vi "DialogRasterCompute.vi"(6 "Mode":bool, 7 "aparCfg in":refnum<class "aparCfg.lvclass">, 10 "Data File Name":string, 11 "Motion64.ini path":path=path "C:/Users/Public/Documents/UCAR/APAR Board Test/SupportFiles/Motion64.ini") -> (1 "Position Array":T1(array[cluster]), 2 "Data File Name out":string, 3 "Cancelled?":bool, 5 "aparCfg out":refnum<class "aparCfg.lvclass">)   [LabVIEW 2017]
doc: "Use this template to create a dialog box with event handling."
uses:
  Classes/VXMCfg/VXMCfg.lvclass
  Classes/aparCfg/aparCfg.lvclass
  <vilib>/Utility/file.llb/Read Delimited Spreadsheet (DBL).vi
panel:
  out "64ModuleConfigs":string[][](table) caption="Configurations for the 64 Modules"
  in  "Polarization":enum16{"Vertical", "Horizontal"}(ring)=enum."Horizontal"
  in  "RF In/Out":enum16{"Tx - RF In", "Rx - RF Out"}(ring)=enum."Rx - RF Out"
  out "Total Points":dbl
  out "TestZT":cluster{"Z mm":dbl, "Horizontal T deg":dbl}
  out "XY Graph for evaluation":cluster{dbl[], dbl[]}[](graph)
  in  "Nyquist, mm":i32=28 caption="Nyquist Sampling Interval, mm" min=1 max=64 step=1
  in  "calculate":bool
  in  "Window dimension":i32=42 caption="Synthetic Window, cm" min=1 max=64 step=1
  in  "Cancel":bool
  in  "OK":bool
  # "Define Raster Positions"
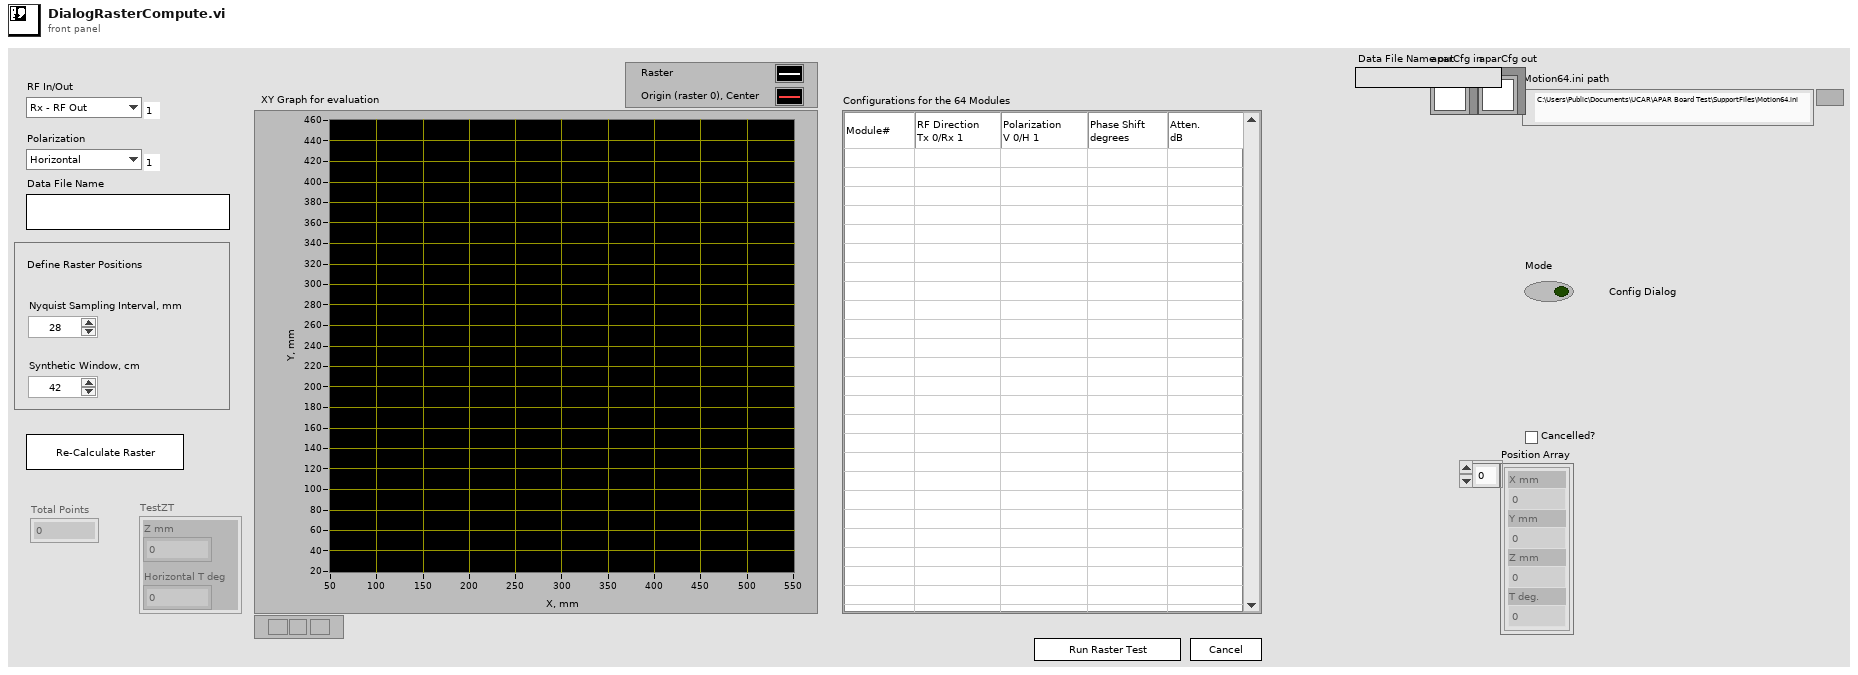
[diagram p1: front panel]
types:
  T1 = cluster{"X mm":dbl, "Y mm":dbl, "Z mm":dbl, "T deg.":dbl}[]
  T2 = typedef "rasterConfig.ctl" = cluster{"Nyquist, mm":dbl, "Window, cm":dbl, "Polarization, V0 H1":T3, "RF Direction Tx0":T4}
  T3 = typedef "PolarizationSelect.ctl" = enum16{"Vertical", "Horizontal"}
  T4 = typedef "RF Direction.ctl" = enum16{"Tx - RF In", "Rx - RF Out"}
  T5 = typedef "sub-syst.n.ctl" = cluster{"Addr":string, "Enable":bool, "X scale eng./step":dbl, "Y scale eng./step":dbl, "Z scale eng./step":dbl, "T scale eng./step":dbl, "X units":string, "Y units":string, "Z units":string, "T units":string, "X Jog":dbl, "Y Jog":dbl, "Z Jog":dbl, "T Jog":dbl, "VXM (1-4)":i32}
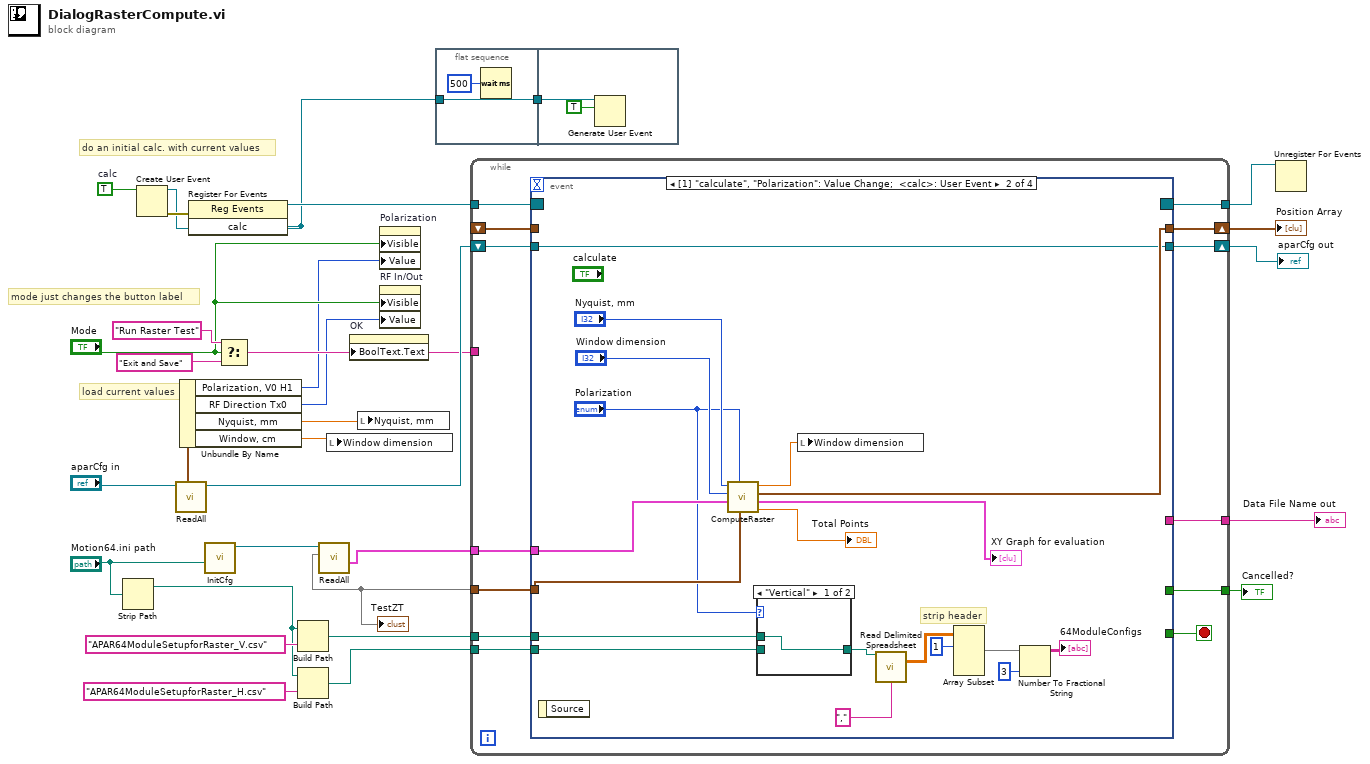
[diagram p0: block diagram]
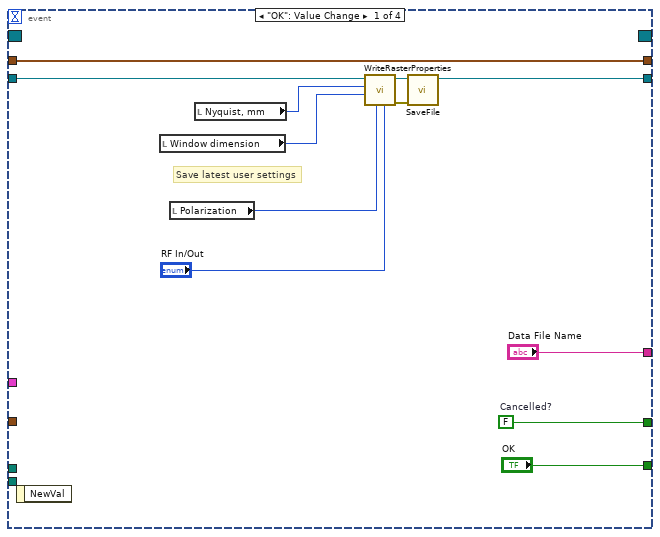
[diagram p2: hidden frame]
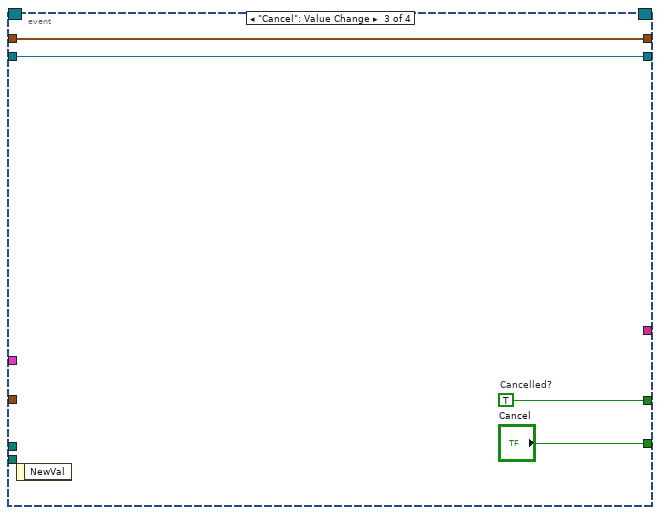
[diagram p4: hidden frame]
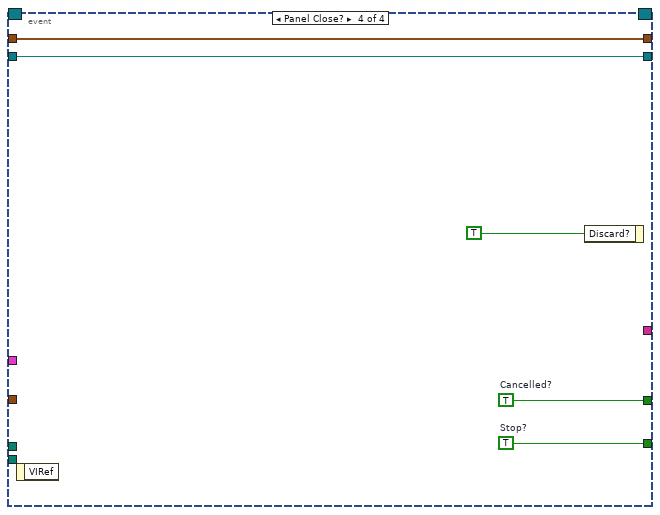
[diagram p5: hidden frame]
diagram:
  w19 = TRUE  # calc
  # "load current values"
  # "do an initial calc. with current values"
  # "mode just changes the button label"
  n1 = Strip Path(path="Motion64.ini path") -> (stripped path=w4:path)  [unwired: 1 out]
  n2 = Create User Event(user event datatype=w19) -> (user event=w15:refnum<user-event>, error out=w18:errorcluster)  [unwired: 1 in]
  n3 = call "ReadAll.vi"("aparCfg in"="aparCfg in") -> ("aparCfg out"=w22:refnum<class "aparCfg.lvclass">, "apar properties.RasterDef"=w25:T2)  [unwired: 4 in, 5 out]
  n4 = Unbundle By Name(w25) -> ("Polarization, V0 H1"=w8:T3, "RF Direction Tx0"=w9:T4, "Nyquist, mm"=w23:dbl, "Window, cm"=w24:dbl)
  n5 = register-events(error in=w18, w15) -> (reference out=w17:refnum<event-registration>)  [unwired: 1 in, 1 out]
  n6 = call "InitCfg.vi"("Cfg File path"="Motion64.ini path") -> ("VXMCfg out"=w29:refnum<class "VXMCfg.lvclass">)  [unwired: 8 in, 2 out]
  n7 = Select(t="Run Raster Test" ("Boolean Text.Text"), s="Mode", f="Exit and Save" ("Boolean Text.Text")) -> (s? t:f=w11:string)
  n8 = Build Path(base path=w4, name or relative path="APAR64ModuleSetupforRaster_V.csv") -> (appended path=w3:path)
  n9 = Build Path(base path=w4, name or relative path="APAR64ModuleSetupforRaster_H.csv") -> (appended path=w2:path)
  n10 = call "ReadAll.vi"("VXMCfg in"=w29) -> ("VXM Properties.sub-syst.3"=w27:T5, 10:w28)  [unwired: 5 in, 4 out]
  "TestZT" <- w28
  n11 = local write "Window dimension"(w24) -> ()
  n12 = property on="OK" class="Bool"("BoolText.Text"=w11) -> ()  [unwired: 2 in, 2 out]
  n13 = local write "Nyquist, mm"(w23) -> ()
  n14 = property on="Polarization" class="Enum (strict)"("Visible"="Mode", "Value"=w8) -> ()  [unwired: 2 in, 2 out]
  n15 = property on="RF In/Out" class="Enum (strict)"("Visible"="Mode", "Value"=w9) -> ()  [unwired: 2 in, 2 out]
  n16 = flat-sequence {
    tunnel: w15 -> [w32]
    tunnel: [w32] -> w14
    tunnel: w14 -> [w33]
    frame #0 {
      n17 = Wait (ms)(milliseconds to wait=u32 500) -> ()  [unwired: 1 out]
    }
    frame #1 {
      n18 = Generate User Event(user event=w33, event data cluster=TRUE ("event data")) -> ()  [unwired: 2 in, 2 out]
    }
  }
  n19 = while {
    tunnel: [w46] -> w30
    tunnel: w28 -> [w45]
    tunnel: w27 -> [w44]
    shift-right: [w43] -> w26
    shift-left: _ -> [w42]
    shift-right: [w40] -> w20
    shift-left: w22 -> [w41]
    tunnel: w17 -> [w39]
    tunnel: [w38] -> w16
    tunnel: w11 -> [_]
    tunnel: w3 -> [w37]
    tunnel: w2 -> [w36]
    tunnel: [w35] -> w1
    stop <- w47 stop-if-true
    n20 = event shown="[1] \"calculate\", \"Polarization\": Value Change;  <calc>: User Event" {
      selector: w39 -> [_ _ _ _]
      dyn-events: [_ _ _ _] -> w38
      timeout: _ -> [_ _ _ _]
      tunnel: ["OK" _ "Cancel" w88] -> w47
      tunnel: [w59 _ w84 w87] -> w46
      tunnel: w45 -> [_ w74 _ _]
      tunnel: w44 -> [_ w78 _ _]
      tunnel: [w57 w75 w82 w86] -> w43
      tunnel: w42 -> [w57 _ w82 w86]
      tunnel: [w50 w70 w81 w85] -> w40
      tunnel: w41 -> [w51 w70 w81 w85]
      tunnel: w37 -> [_ w65 _ _]
      tunnel: w36 -> [_ w64 _ _]
      tunnel: ["Data File Name" _ _ _] -> w35
      event "OK": Value Change {
        w59 = FALSE  # Cancelled?
        # "Save latest user settings"
        n21 = event-data() -> ()  [unwired: 1 in, 1 out]
        n22 = local read "Window dimension"() -> (w54:i32)
        n23 = local read "Polarization"() -> (w49:enum16{"Vertical", "Horizontal"})
        n24 = local read "Nyquist, mm"() -> (w55:i32)
        n25 = call "WriteRasterProperties.vi"("Direction Tx0"="RF In/Out", "Polarization, V0 H1"=w49, "Window, cm"=w54, "Nyquist, mm"=w55, "aparCfg in"=w51) -> ("error out"=w56:errorcluster, "aparCfg out"=w52:refnum<class "aparCfg.lvclass">)  [unwired: 5 in]
        n26 = call "SaveFile.vi"("error in (no error)"=w56, "aparCfg in"=w52) -> ("aparCfg out"=w50:refnum<class "aparCfg.lvclass">)  [unwired: 8 in, 1 out]
      }
      event "calculate", "Polarization": Value Change; User Event {
        # "strip header"
        n27 = event-data() -> ()  [unwired: 1 in, 1 out]
        n28 = call "ComputeRaster.vi"("TestZT"=w74, "Polarization, V0 H1"="Polarization", "Position Array in"=w78, "Window dimension"="Window dimension", "Nyquist, mm"="Nyquist, mm") -> ("Total points"=→"Total Points":dbl, "XY Graph for evaluation"=→"XY Graph for evaluation":cluster{dbl[], dbl[]}[], "Position Array out"=w75:T1, "Window adjusted, cm"=w77:dbl)  [unwired: 3 in]
        n29 = case shown="\"Vertical\"" "Polarization" {
          tunnel: w64 -> [_ w80]
          tunnel: [w79 w80] -> w68
          tunnel: w65 -> [w79 _]
          frame "Vertical" {
          }
          frame "Horizontal", Default {
          }
        }
        n30 = local write "Window dimension"(w77) -> ()
        n31 = call-poly <vilib>:"Read Delimited Spreadsheet.vi"("file path (dialog if empty)"=w68, "delimiter (\\t)"="," ("delimiter (\\t)")) -> ("all rows"=w69:dbl[][])  [unwired: 8 in, 5 out]
        n32 = Array Subset(array=w69, index (row)=1 ("index")) -> (w63:dbl[][])  [unwired: 3 in]
        n33 = Number To Fractional String(number=w63, precision (6)=i16 3) -> (F-format string=→"64ModuleConfigs":string[][])  [unwired: 2 in]
      }
      event "Cancel": Value Change {
        w84 = TRUE  # Cancelled?
        n34 = event-data() -> ()  [unwired: 1 in, 1 out]
      }
      event Panel Close? {
        w87 = TRUE  # Cancelled?
        w88 = TRUE  # Stop?
        n35 = event-data() -> ()  [unwired: 1 in, 1 out]
        n36 = event-data("Discard?"=TRUE) -> ()  [unwired: 1 in, 1 out]
      }
    }
  }
  "Cancelled?" <- w30
  "Position Array" <- w26
  "aparCfg out" <- w20
  "Data File Name out" <- w1
  n37 = Unregister For Events(event registration refnum=w16) -> ()  [unwired: 1 in, 1 out]
